vi "Calc speed given dist quadratic.vi"(0 "Distance from dest":dbl=500.0, 5 "Min dist for movement":dbl=50.0, 9 "min speed":dbl=0.3, 11 "error in (no error)":errorcluster, 12 "max speed":dbl=4.0) -> (14 "Speed":dbl, 15 "error out":errorcluster)   [LabVIEW 2016]
panel:
  in  "Distance at speed 4":dbl=300.0
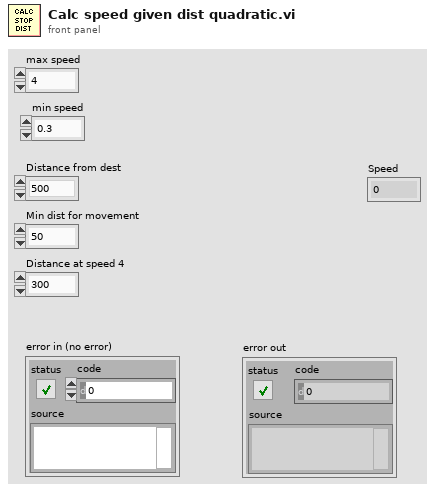
[diagram p1: front panel]
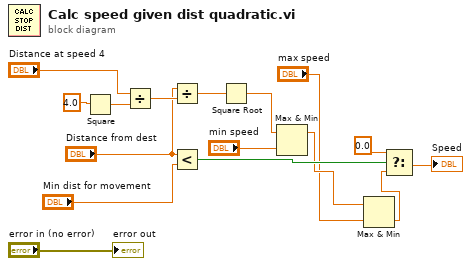
[diagram p0: block diagram]
diagram:
  n1 = Square(x=4.0) -> (x^2=w15:dbl)
  n2 = Divide(x="Distance at speed 4", y=w15) -> (x/y=w12:dbl)
  n3 = Divide(x="Distance from dest", y=w12) -> (x/y=w11:dbl)
  n4 = Less?(x="Distance from dest", y="Min dist for movement") -> (x < y?=w6:bool)
  n5 = Square Root(x=w11) -> (sqrt(x)=w10:dbl)
  n6 = Max & Min(x=w10, y="min speed") -> (max(x,y)=w3:dbl)  [unwired: 1 out]
  n7 = Max & Min(x=w3, y="max speed") -> (min(x,y)=w1:dbl)  [unwired: 1 out]
  n8 = Select(t=0.0, s=w6, f=w1) -> (s? t:f=→"Speed":dbl)
  "error out" <- "error in (no error)"
